vi "LEBITplc.PubSetServices.vi"(0 "i ref in":refnum<vi>, 2 "i attribute in":T1, 5 "error in":errorcluster) -> (14 "i ref out":refnum<vi>, 16 "i attribute out":T1, 17 "SetValueServiceID":i32[](array[numeric]), 19 "error out":errorcluster)   [LabVIEW 2014, in "LEBITplc.lvlib"]
uses:
  LEBITplc.lvlib
  CS_Core/CAEObj/CAEObj.event definition.ctl
  CS_Core/BaseProcess/BaseProcess.event definition.ctl
  CS_Core/BaseProcess/BaseProcess.descriptor string definition.ctl
  LEBITplc.i attribute.ctl
  CSlibraries/UtilityLib/UtilityLib.valueStatus.ctl
  CSlibraries/UtilityLib/UtilityLib.lvlib
  CS_Core/CSSystem/CoreLib/CoreLib.lvlib
  CSlibraries-extern/DimLVEvent/LVDimInterface/LVDimInterface.lvlib
  CS_Core/BaseProcess/BaseProcess.lvlib
  CS_Core/CAEObj/CAEObj.lvlib
panel:
  in  "event definition":T2
  in  "CAEEvtDef":T3
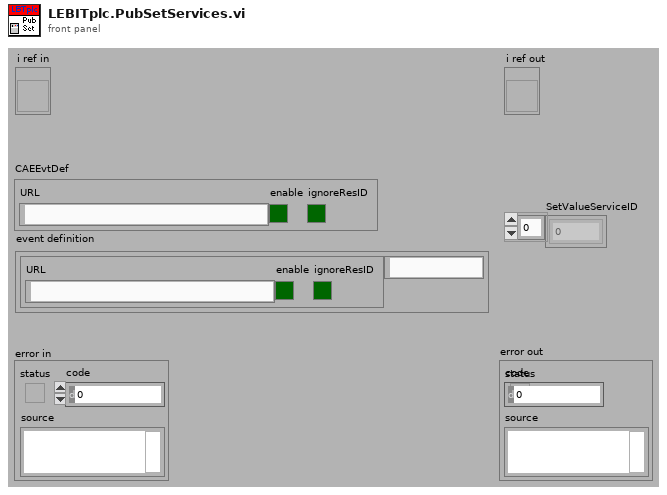
[diagram p1: front panel]
types:
  T1 = typedef "LEBITplc.lvlib/LEBITplc.i attribute.ctl" = cluster{"LLFLocation":string, "SetFileLocation":string, "nickNames":string[], "setValuePLCServiceID":i32[], "GUIServiceID":i32[], "monValuePLC":string[], "SetValueServiceID":i32[], "MonValueServiceID":i32[], "SetValue":dbl[][], "SetValueMin":dbl[], "SetValueMax":dbl[], "SetValueInfoServiceID":i32[], "GUINames":string[], "ListOfBases":string[], "Scale":dbl[], "Offset":dbl[], "setValuePLC":string[], "BaseName":string[], "ScaleServiceID":i32[], "OffsetServiceID":i32[], "AllPLCValues":string[], "CondSpecialArray":string[][], "CondSpecialIndex":i32[], "CondSpecialMonValue":dbl[], "RecentlyChanged":i32[], "SetFileLocationID":i32, "Dependent-Monitors":string[][], "LastLoadedFiles":string[], "IonGuideCalibLocation":string, "Monitor Dependent":string[], "Special":string[], "PLC?":bool[], "Start Date":string, "ListOfBasesServiceID":i32, "SETRA VISA resource":refnum<visa-resource-name>}
  T2 = typedef "BaseProcess.lvlib/BaseProcess.event definition.ctl" = cluster{"CAEEvtDef":T3, "Data Descriptor":T4}
  T3 = typedef "CAEObj.lvlib/CAEObj.event definition.ctl" = cluster{"URL":string, "enable":bool, "ignoreResID":bool}
  T4 = typedef "BaseProcess.lvlib/BaseProcess.descriptor string definition.ctl" = string
  T5 = typedef "UtilityLib.lvlib/UtilityLib.valueStatus.ctl" = enum16{"no info available", "stand by/off", "on", "warning", "alarm/malfunction", "not implemented", "user action required", "important information", "system default", "control default", "indicator default", "button default"}
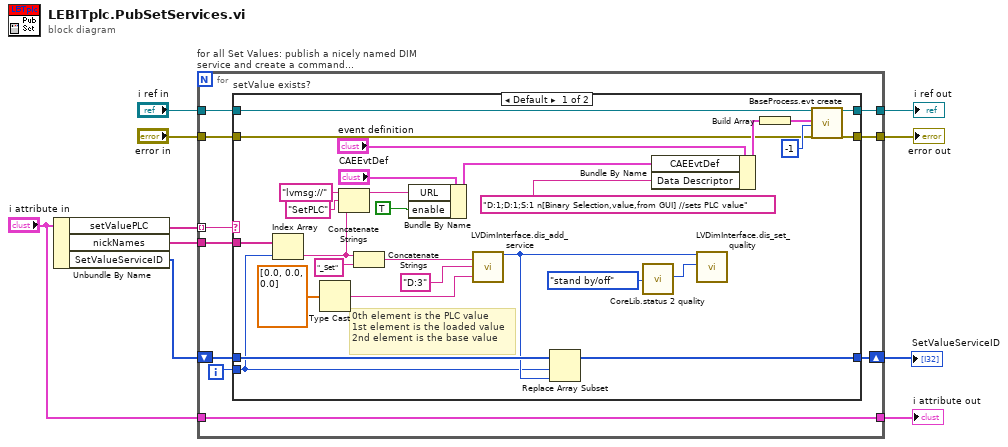
[diagram p0: block diagram]
diagram:
  n1 = Unbundle By Name("i attribute in") -> ("setValuePLC"=w4:string[], "nickNames"=w5:string[], "SetValueServiceID"=w1:i32[])
  n2 = for "for all Set Values: publish a nicely named DIM service and create a command..." {
    tunnel: w4 -> [w20] mode=indexing
    tunnel: w5 -> [w19]
    shift-right: [w16] -> w10
    shift-left: w1 -> [w17]
    tunnel: "i ref in" -> [w15]
    tunnel: "error in" -> [w14]
    tunnel: [w13] -> w9
    tunnel: [w12] -> w8
    tunnel: "i attribute in" -> [w11]
    tunnel: [w11] -> w2
    i -> [w18]
    n3 = case "setValue exists?" shown="Default" w20 {
      tunnel: w19 -> [w46 _]
      tunnel: w18 -> [w23 _]
      tunnel: w17 -> [w44 w51]
      tunnel: [w43 w51] -> w16
      tunnel: w15 -> [w42 w50]
      tunnel: w14 -> [w29 w49]
      tunnel: [w28 w49] -> w13
      tunnel: [w27 w50] -> w12
      frame Default {
        # "0th element is the PLC value\n1st element is the loaded value\n2nd element is the base value"
        n4 = Index Array(array=w46, index=w23) -> (element=w34:string)
        n5 = Type Cast(x=dbl[] [0.0, 0.0, 0.0]) -> (*(type *) &x=w45:string)  [unwired: 1 in]
        n6 = Concatenate Strings("lvmsg://" ("string"), "SetPLC" ("string"), w34) -> (w37:string)
        n7 = Concatenate Strings(w34, "_Set" ("string")) -> (w47:string)
        n8 = Bundle By Name(cluster="CAEEvtDef", "URL"=w37, "enable"=TRUE) -> (w38:T3)
        n9 = call "LVDimInterface.dis_add_service.vi"("serviceName"=w47, "typeDescriptor"="D:3", "data"=w45) -> ("my_serviceID"=w25:i32)  [unwired: 15 in, 1 out]
        n10 = Replace Array Subset(array=w44, new element=w25, index=w23) -> (w43:i32[])
        n11 = call "CoreLib.status 2 quality.vi"("valueStatus"=UtilityLib.valueStatus."stand by/off") -> ("quality"=w24:i32)  [unwired: 18 in]
        n12 = Bundle By Name(cluster="event definition", "CAEEvtDef"=w38, "Data Descriptor"="D:1;D:1;S:1 n[Binary Selection,value,from GUI] //sets PLC value" ("string")) -> (w31:T2)
        n13 = call "LVDimInterface.dis_set_quality.vi"("my_serviceID"=w25, "quality"=w24) -> ()  [unwired: 16 in, 2 out]
        n14 = Build Array(w31) -> (w30:T2[])
        n15 = call "BaseProcess.evt create.vi"("i ref in"=w42, "newEvents"=w30, "ms timeout (10000)"=-1, "error in (no error)"=w29) -> ("i ref out"=w27:refnum<vi>, "error out"=w28:errorcluster)  [unwired: 12 in, 2 out]
      }
      frame "" {
      }
    }
  }
  "SetValueServiceID" <- w10
  "error out" <- w9
  "i ref out" <- w8
  "i attribute out" <- w2
